vi "Log.vi"(10 "Log Packet":T1, 11 "String Log Sink in":refnum<class "String Log Sink.lvclass">) -> (0 "error out":errorcluster, 3 "String Log Sink out":refnum<class "String Log Sink.lvclass">)   [LabVIEW 2019, in "String Log Sink.lvclass"]
uses:
  String Log Sink.lvclass
  Composed Log/Types/Log Packet.ctl
  Composed Log/Types/Log Level.ctl
  Composed Log/Composed Log.lvlib
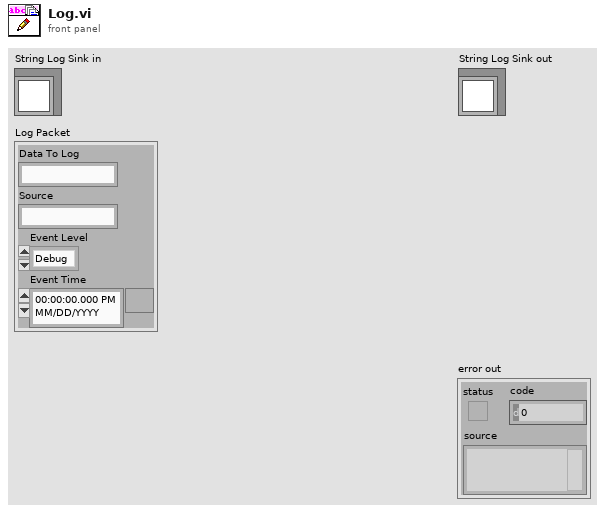
[diagram p1: front panel]
types:
  T1 = typedef "Composed Log.lvlib/Log Packet.ctl" = cluster{"Data To Log":string, "Source":string, "Event Level":T2, "Event Time":timestamp}
  T2 = typedef "Composed Log.lvlib/Log Level.ctl" = enum16{"Debug", "Info", "Warning", "Error", "Critical"}
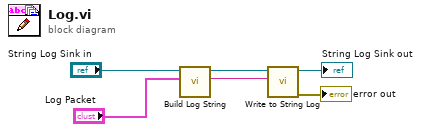
[diagram p0: block diagram]
diagram:
  n1 = call-dynamic "Build Log String.vi"("Log Packet"="Log Packet", "String Log Sink in"="String Log Sink in") -> ("Log Entry"=w2:string, "String Log Sink out"=w3:refnum<class "String Log Sink.lvclass">)  [unwired: 8 in]
  n2 = call-dynamic "Write to String Log.vi"("String to Log"=w2, "String Log Sink in"=w3) -> ("error out"=→"error out":errorcluster, "String Log Sink out"=→"String Log Sink out":refnum<class "String Log Sink.lvclass">)  [unwired: 8 in]
